vi "Set ToolTip.vi"(8 "error in":errorcluster, 11 "Cell in":refnum<class "Cell.lvclass">) -> (0 "error out":errorcluster, 3 "Cell out":refnum<class "Cell.lvclass">)   [LabVIEW 2024, in "SourceGrid.lvlib" / "Cell.lvclass"]
uses:
  Cell.lvclass
  Cell.lvclass/Cell.ctl
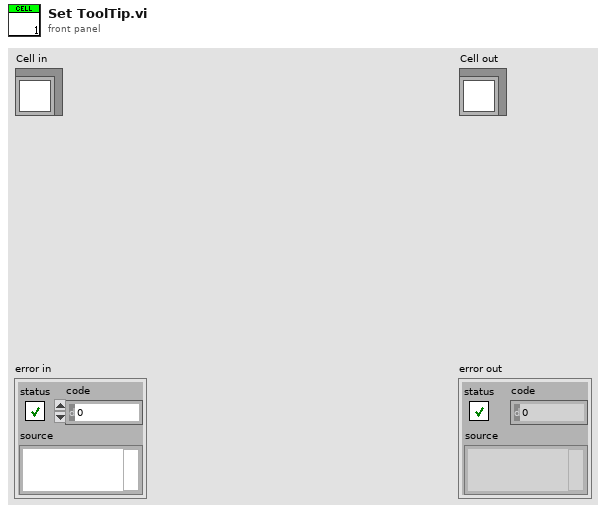
[diagram p1: front panel]
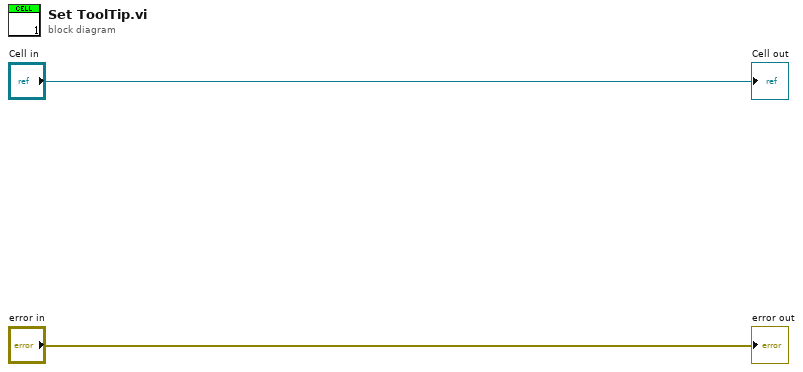
[diagram p0: block diagram]
diagram:
  "error out" <- "error in"
  "Cell out" <- "Cell in"
